vi "Top Level FPGA_LEDdebug.vi"() -> ()   [LabVIEW 2012]
uses:
  <vilib>/Platform/TimedLoop/XDataNode/timing_clust.ctl
  <vilib>/Platform/TimedLoop/XDataNode/nitl_modes.ctl
  <vilib>/Platform/TimedLoop/XDataNode/wakeup.ctl
  <vilib>/rvi/DataTransferAndStorage/Container/Common/niFpgaContainerMetaDataKey.ctl
  <vilib>/rvi/DataTransferAndStorage/Container/Common/niFpgaContainerState.ctl
  <vilib>/rvi/DataTransferAndStorage/Container/Common/niFpgaDataTypeControl.ctl
  <vilib>/rvi/DataTransferAndStorage/Container/Common/niFpgaContainerImplementationControl.ctl
  <vilib>/rvi/DataTransferAndStorage/Container/Common/niFpgaContainerArbitrationOptionsControl.ctl
  <vilib>/rvi/DataTransferAndStorage/Container/Common/niFpgaTransferTypeControl.ctl
  <vilib>/rvi/DataTransferAndStorage/Container/Common/niFpgaContainerInitializationParameters.ctl
  <vilib>/rvi/Memory/Memory_Types/niFpgaMemoryInterfaceConfiguration.ctl
  <vilib>/rvi/FIFO/Fifo_Types/niFpgaFifoControlLogicControl.ctl
  <vilib>/rvi/eio/common/nirviEmuTemplateMethod_errors.vi
  <vilib>/rvi/FIFO/Fifo_Resource/nirvififoEmulationSetSize.vi
  <vilib>/rvi/DataTransferAndStorage/Container/Common/niFpgaContainerGetUniqueNameForEmu.vi
  <vilib>/rvi/Emulation/niFpgaSctlEmulationRegisterWithScheduler.vi
  <vilib>/rvi/Emulation/niFpgaSctlEmulationScheduler.vi
  <vilib>/rvi/Emulation/niFpgaSctlEmulationFifoFullMgr.vi
  <vilib>/rvi/errors/niFpgaSetErrorForExecOnDevCompSimple.vi
  <vilib>/rvi/eio/common/nirviEmuReportErrorAndStop.vi
  <vilib>/rvi/Memory/Memory_Emulation/nirvimemoryEmulationManagerCache_GetValue.vi
  <vilib>/rvi/Memory/Memory_Emulation/niFpgaMemoryEmulationValidateCache.vi
  <vilib>/rvi/Memory/Memory_Emulation/nirvimemoryEmulationManagerCache_InsertValue.vi
  <vilib>/rvi/Memory/Memory_Emulation/nirvimemoryEmulationManagerCache_SetValue.vi
  <vilib>/rvi/Emulation/niFpgaSctlEmulationResourceMgr.vi
  <vilib>/rvi/Memory/Memory_Emulation/niFpgaMemoryEmulationCacheClearOnFirstRun.vi
  <vilib>/rvi/Memory/Memory_Emulation/nirvimemoryEmulationManagerCache_MakeExclusive.vi
  <vilib>/rvi/Memory/Memory_Emulation/nirvimemoryEmulationManagerCache_ReleaseExclusive.vi
  <vilib>/Utility/error.llb/Clear Errors.vi
  <vilib>/rvi/DataTransferAndStorage/Container/Common/niFpgaContainerSetEmuInfo.vi
  <vilib>/eio/EIONode/EIONode.xnode
  <vilib>/Platform/TimedLoop/XDataNode/XDataNode.xnode
  <vilib>/rvi/DataTransferAndStorage/Container/XNode/niFpgaContainer.xnode
  <vilib>/rvi/FIFO/Fifo_Resource/nirvififoEmulationClear.vi
  <vilib>/rvi/FIFO/Fifo_Resource/nirvififoEmulationRead.vi
  <vilib>/rvi/DataTransferAndStorage/Register/Emulation/niFpgaRegisterEmulation.vi
  <vilib>/rvi/Memory/Memory_Emulation/nirvimemoryEmulation.vi
  <vilib>/rvi/FIFO/Fifo_Resource/nirvififoEmulationWrite.vi
  <vilib>/rvi/LocalResourceManager/LocalResourceManager.xnode
  <vilib>/Platform/TimedLoop/XDataNode/XDNodeRunTimeDep.lvlib
panel:
  out "Total number of pulses sent":u64
  out "IO Module\\ADC Error A":bool
  out "IO Module\\ADC Error B":bool
  out "IO Module\\Pll Unlocked":bool
  out "Exited cleanly?":bool
  in  "Stop FPGA and exit":bool
  in  "Record Size only data":u32=95
  in  "show_trigger_position_for_debugging":bool
  out "DMA FIFO Timed Out?":bool
  in  "circular buffer length":u32=1000
  in  "location":i16(ring) items=["Purdue", "NIKHEF", "Zurich", "???"]
  in  "Trigger 0":i16=4000
  in  "Trigger 1":i16=4000
  in  "Trigger 2":i16=4000
  in  "Trigger 3":i16=4000
  in  "Trigger 4":i16=4000
  in  "Trigger 5":i16=4000
  in  "Trigger 6":i16=4000
  in  "Trigger 7":i16=4000
  in  "# of pretrigger":u32=20
  in  "initial value":u64
  in  "channel 0 on/off":bool
  in  "channel 2 on/off":bool
  in  "channel 1 on/off":bool
  in  "channel 3 on/off":bool
  in  "channel 4 on/off":bool
  in  "channel 5 on/off":bool
  in  "channel 6 on/off":bool
  in  "channel 7 on/off":bool
  in  "Testpulse duration (20 ns ticks)":u32=1
  in  "Testpulse Separation (20 ns ticks)":u32=50000
  in  "Testpulse Time Delay (20 ns ticks)":u32=15
  out "Timestamp":u64
  in  "Testpulser On/Off":bool
  out "Init Done":bool
  out "Initialize Flush DMA FIFO":bool
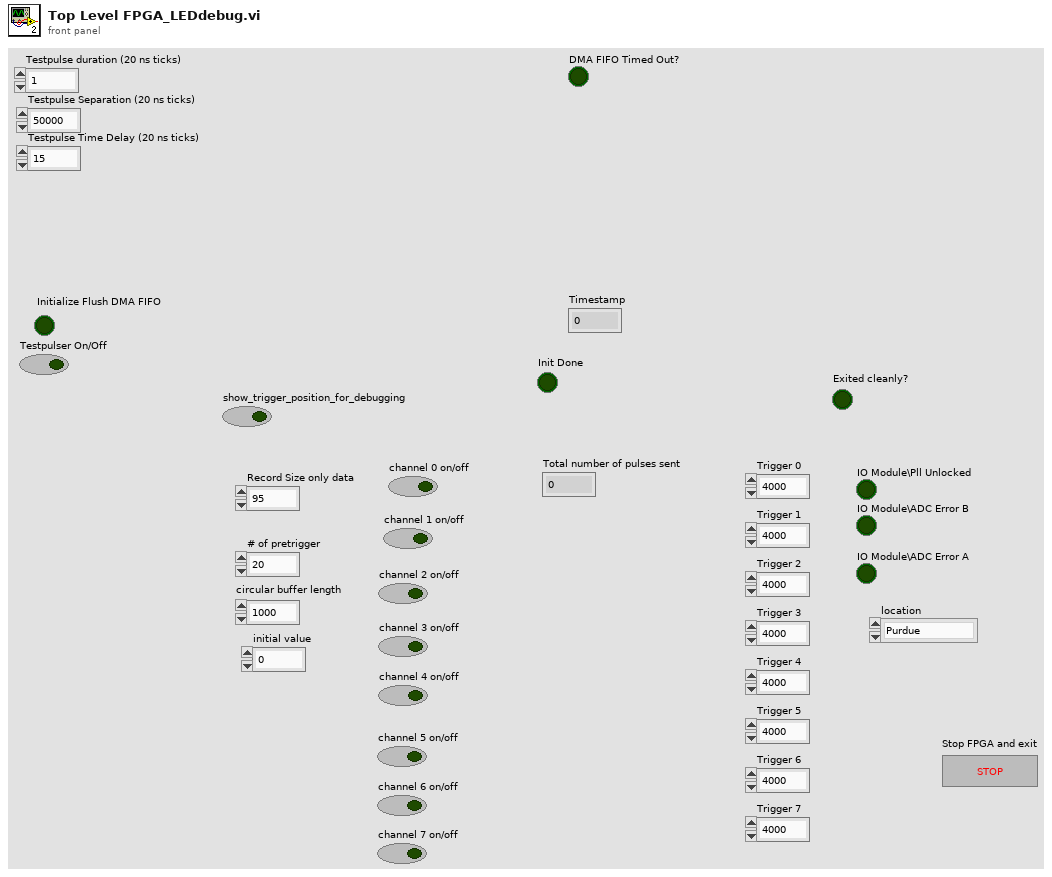
[diagram p1: front panel]
types:
  T1 = typedef "XDNodeRunTimeDep.lvlib/timing_clust.ctl" = cluster{"Expected End [f-1]":u64, "Actual End [f-1]":u64, "Finished Late? [f-1]":bool, "Expected End [i-1]":u64, "Actual End [i-1]":u64, "Finished Late? [i-1]":bool, "Expected Start [i]":u64, "Actual Start [i]":u64, "Expected Start [f]":u64, "Actual Start [f]":u64, "Source Name":string, "Structure Name":string, "Period":i64, "Deadline":i64, "Offset":i64, "Start":i64, "Priority":i32, "Timeout":i32, "Mode":T2, "Wakeup Reason":T3, "Error":errorcluster, "Source Type":string, "Secondary Source Type":string, "Global End Time":u64, "Global Start Time":u64, "Frame Duration":u64, "Iteration Duration":u64, "Assigned CPU":i32, "I/O Scan Engine Mode":u32}
  T2 = typedef "XDNodeRunTimeDep.lvlib/nitl_modes.ctl" = enum32{"No Change", "Process missed periods, maintain original phase", "Discard missed periods, maintain original phase", "Process missed periods, ignore original phase", "Discard missed periods, ignore original phase"}
  T3 = typedef "XDNodeRunTimeDep.lvlib/wakeup.ctl" = enum32{"Normal", "Aborted", "Asynchronous wakeup", "Timing source error", "Timed loop error", "Timeout"}
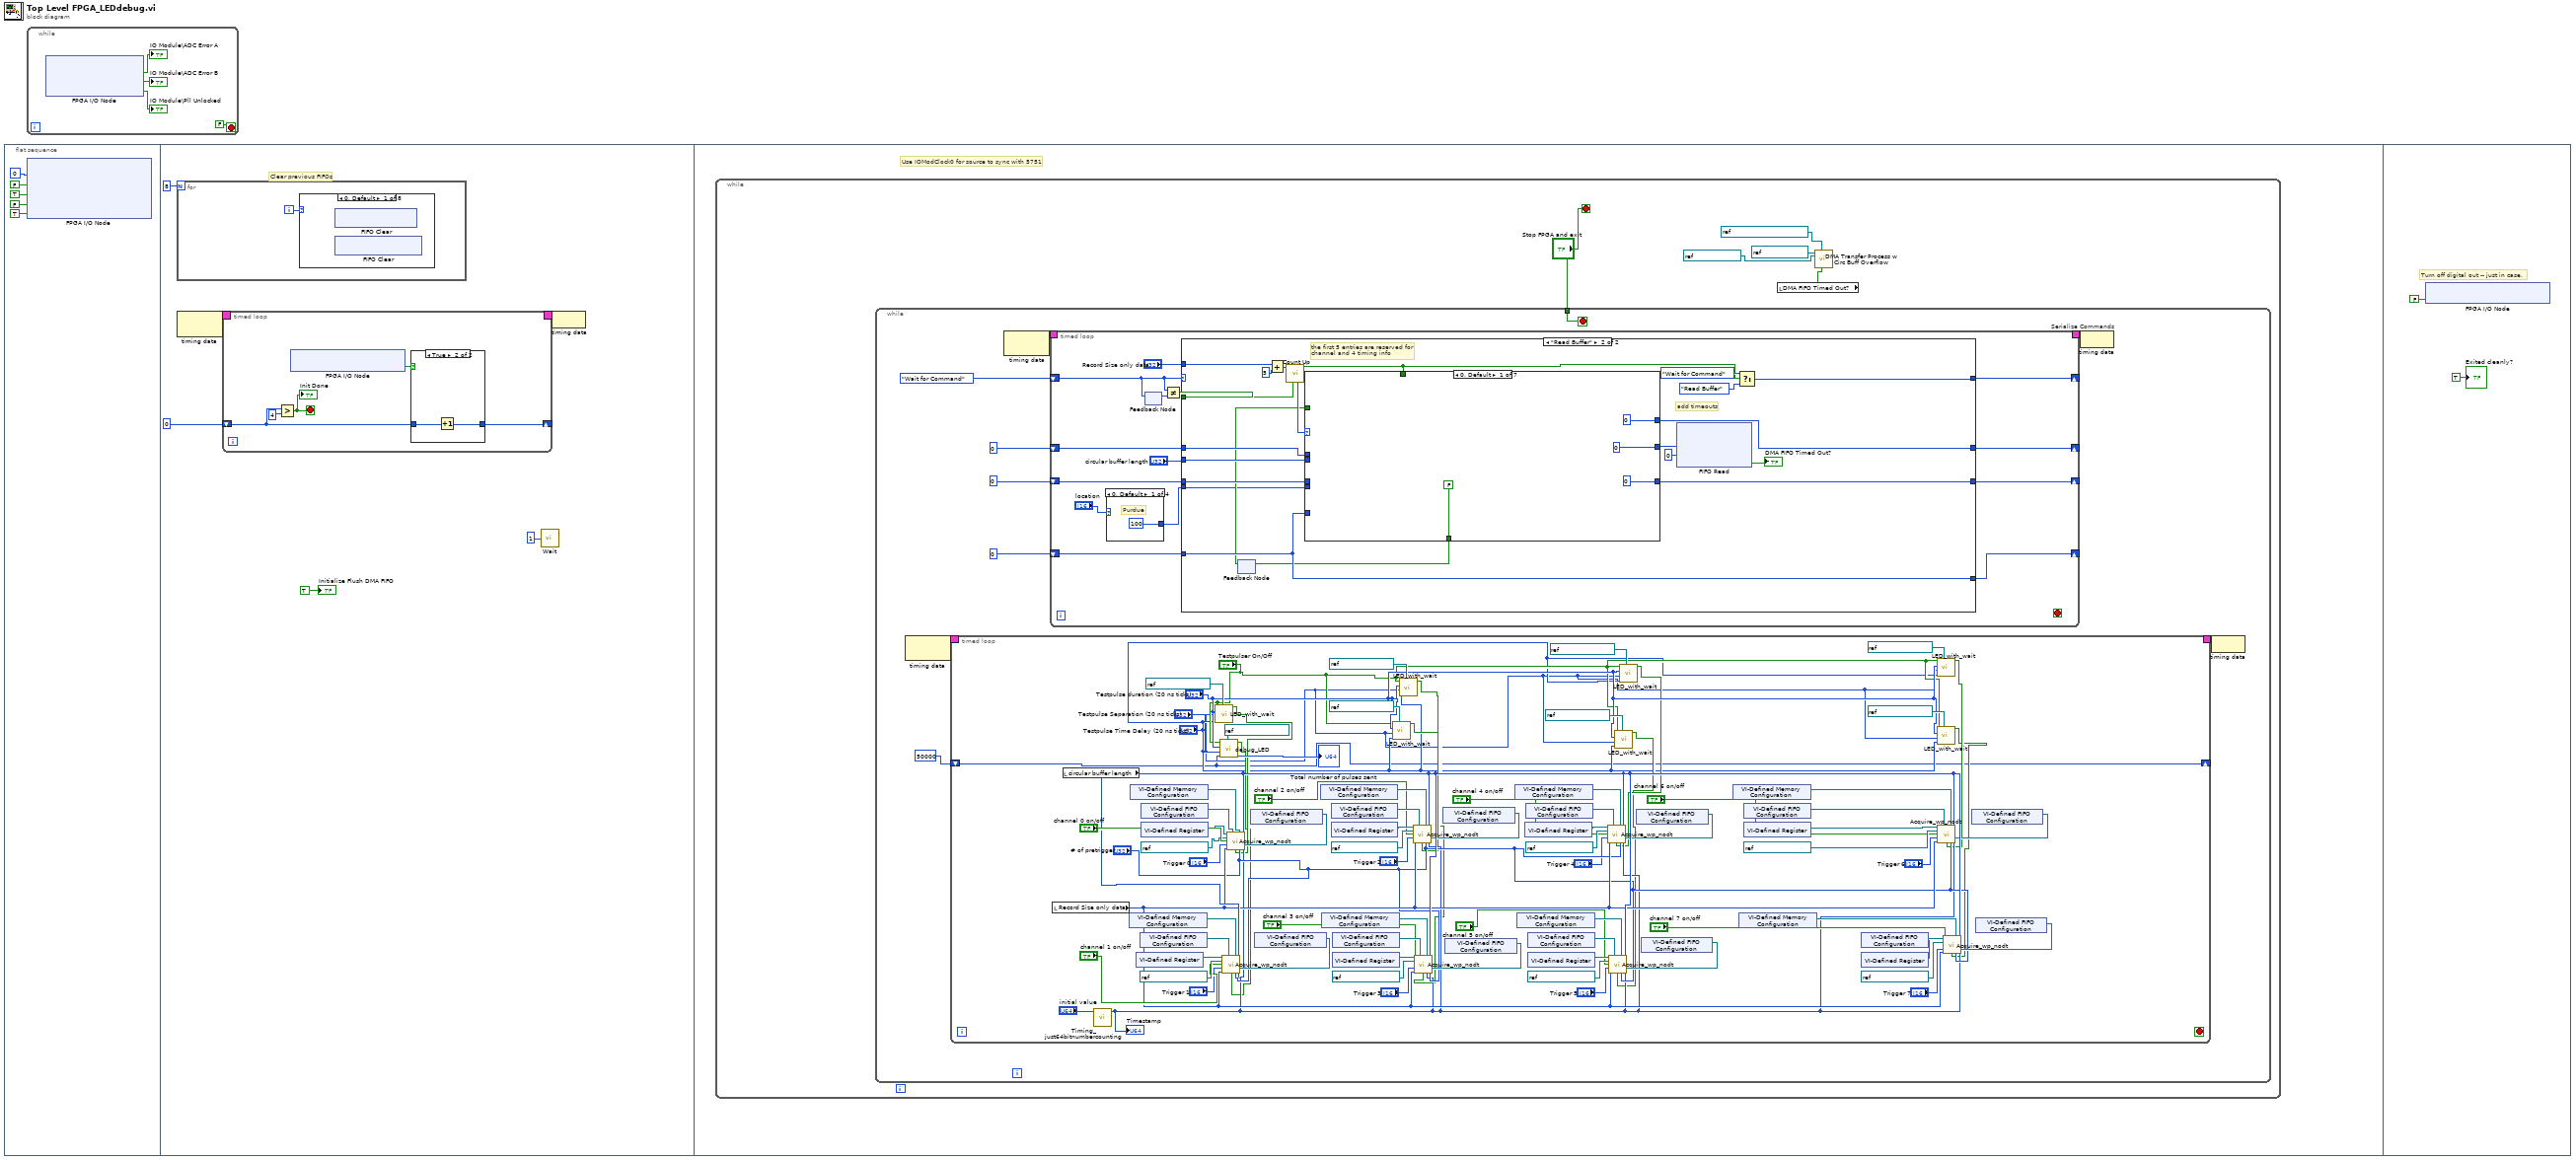
[diagram p0: block diagram]
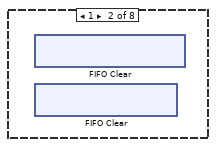
[diagram p2: hidden frame]
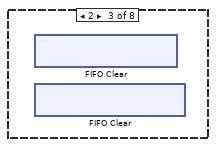
[diagram p3: hidden frame]
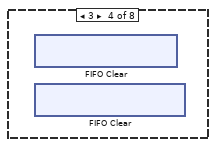
[diagram p4: hidden frame]
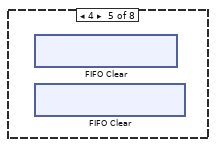
[diagram p5: hidden frame]
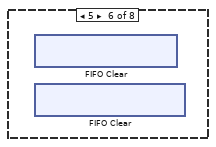
[diagram p6: hidden frame]
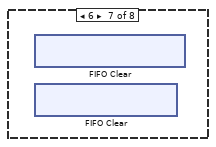
[diagram p7: hidden frame]
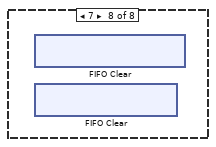
[diagram p8: hidden frame]
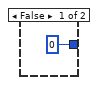
[diagram p9: hidden frame]
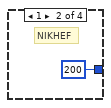
[diagram p10: hidden frame]
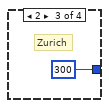
[diagram p11: hidden frame]
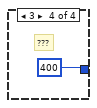
[diagram p12: hidden frame]
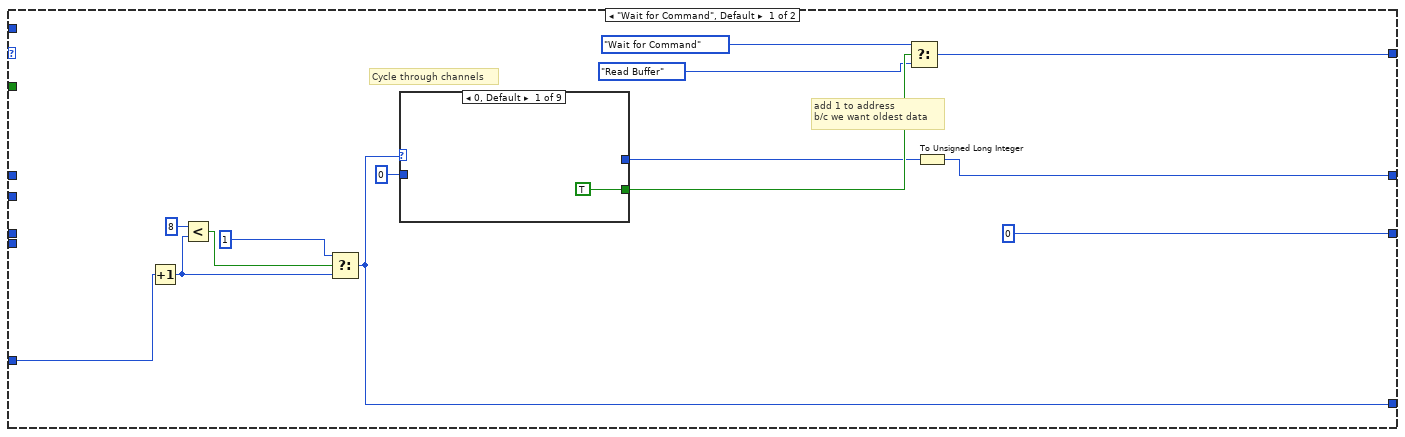
[diagram p13: hidden frame]
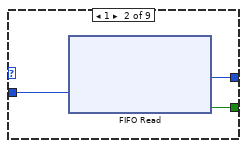
[diagram p14: hidden frame]
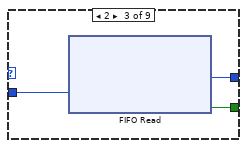
[diagram p15: hidden frame]
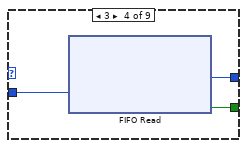
[diagram p16: hidden frame]
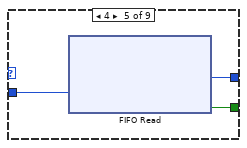
[diagram p17: hidden frame]
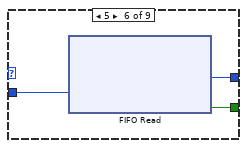
[diagram p18: hidden frame]
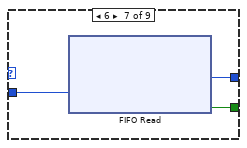
[diagram p19: hidden frame]
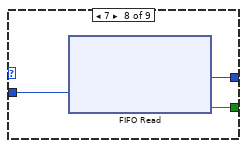
[diagram p20: hidden frame]
diagram:
  n1 = flat-sequence {
    frame #0 {
      n2 = xnode "FPGA I/O Node"("IO Module\\Sample Clock Select"=u8 0 ("IO Module\\Sample Clock Select"), "IO Module\\Force Initialization"=FALSE ("IO Module\\Force Initialization"), "IO Module\\Force Initialization"=TRUE ("IO Module\\Force Initialization"), "IO Module\\Force Initialization"=FALSE ("IO Module\\Force Initialization"), "IO Module\\Digital Output Enable"=TRUE ("IO Module\\Digital Output Enable")) -> ()  [unwired: 5 in, 5 out]
    }
    frame #1 {
      # "Clear previous FIFOs"
      n3 = for {
        N: 8 -> [_]
        i -> [w12]
        n4 = case shown="0, Default" w12 {
          frame 0, Default {
            n5 = xnode ("FIFO Clear")() -> ()  [unwired: 1 in, 1 out]
            n6 = xnode ("FIFO Clear")() -> ()  [unwired: 1 in, 1 out]
          }
          frame 1 {
            n7 = xnode ("FIFO Clear")() -> ()  [unwired: 1 in, 1 out]
            n8 = xnode ("FIFO Clear")() -> ()  [unwired: 1 in, 1 out]
          }
          frame 2 {
            n9 = xnode ("FIFO Clear")() -> ()  [unwired: 1 in, 1 out]
            n10 = xnode ("FIFO Clear")() -> ()  [unwired: 1 in, 1 out]
          }
          frame 3 {
            n11 = xnode ("FIFO Clear")() -> ()  [unwired: 1 in, 1 out]
            n12 = xnode ("FIFO Clear")() -> ()  [unwired: 1 in, 1 out]
          }
          frame 4 {
            n13 = xnode ("FIFO Clear")() -> ()  [unwired: 1 in, 1 out]
            n14 = xnode ("FIFO Clear")() -> ()  [unwired: 1 in, 1 out]
          }
          frame 5 {
            n15 = xnode ("FIFO Clear")() -> ()  [unwired: 1 in, 1 out]
            n16 = xnode ("FIFO Clear")() -> ()  [unwired: 1 in, 1 out]
          }
          frame 6 {
            n17 = xnode ("FIFO Clear")() -> ()  [unwired: 1 in, 1 out]
            n18 = xnode ("FIFO Clear")() -> ()  [unwired: 1 in, 1 out]
          }
          frame 7 {
            n19 = xnode ("FIFO Clear")() -> ()  [unwired: 1 in, 1 out]
            n20 = xnode ("FIFO Clear")() -> ()  [unwired: 1 in, 1 out]
          }
        }
      }
      n21 = node-c288() -> (w11:T1)  [unwired: 1 in]
      n22 = timed-loop {
        shift-right: [w16] -> _
        shift-left: u16 0 -> [w15]
        timing: w11 -> [_]
        timing-out: [_] -> w10
        stop <- w13 stop-if-true
        n23 = Greater?(x=w15, y=u16 4) -> (0:w13:bool)
        "Init Done" <- w13
        n24 = xnode "FPGA I/O Node"() -> ("IO Module\\Initialization Done"=w17:bool)  [unwired: 1 in, 1 out]
        n25 = case shown="True" w17 {
          tunnel: [u16 0 w20] -> w16
          tunnel: w15 -> [_ w19]
          frame False {
          }
          frame True {
            n26 = Increment(x=w19) -> (x+1=w20:u16)
          }
        }
      }
      n27 = call "Wait"("Count(mSec)"=u32 1) -> ()  [unwired: 1 out]
      n28 = node-c288(w10) -> ()
      "Initialize Flush DMA FIFO" <- TRUE ("Initialize Flush DMA FIFO")
    }
    frame #2 {
      # "Use IOModClock0 for source to sync with 5751"
      n29 = while {
        stop <- "Stop FPGA and exit" stop-if-true
        n30 = while {
          tunnel: "Stop FPGA and exit" -> [w31]
          stop <- w31 stop-if-true
          n31 = node-c288() -> (w37:T1)  [unwired: 1 in]
          n32 = timed-loop {
            timing: w37 -> [_]
            timing-out: [_] -> w36
            shift-right: [w40] -> _
            shift-left: u32 50000 ("Testpulse Separation (20 ns ticks) 3") -> [w40]
            stop <- _ stop-if-true
            n33 = local read "Record Size only data"() -> (w82:u32)
            n34 = local read "circular buffer length"() -> (w83:u32)
            n35 = call "Timing_just64bitnumbercounting.vi"("initial value"="initial value") -> ("x+1"=w54:u64)  [unwired: 10 in]
            "Timestamp" <- w54
            n36 = xnode "VI-Defined Memory Configuration"() -> ("Memory Out"=w122:refnum<k21>)
            n37 = xnode "VI-Defined Memory Configuration"() -> ("Memory Out"=w84:refnum<k21>)
            n38 = xnode "VI-Defined Register"() -> ("Register Out"=w78:refnum<k21>)
            n39 = xnode "VI-Defined FIFO Configuration"() -> ("FIFO Out"=w121:refnum<k21>)
            n40 = xnode "VI-Defined FIFO Configuration"() -> ("FIFO Out"=w85:refnum<k21>)
            n41 = xnode "VI-Defined Register"() -> ("Register Out"=w79:refnum<k21>)
            n42 = call "LED_with_wait.vi"("FPGA I/O In"=refnum<k21> "IO Module\\D0 0", "Testpulse Time Delay (20 ns ticks)"="Testpulse Time Delay (20 ns ticks)", "Testpulse Separation (20 ns ticks)"="Testpulse Separation (20 ns ticks)", "Testpulse duration (20 ns ticks)"="Testpulse duration (20 ns ticks)", "Testpulser On/Off"="Testpulser On/Off") -> ("Is Test Pulse?"=w50:bool)  [unwired: 4 in, 2 out]
            n43 = call "debug_LED.vi"("FPGA I/O In"=refnum<k21> "IO Module\\D0 1", "Test pulse separation (20 ns ticks)"=w40, "Testpulse Time Delay (20 ns ticks)"="Testpulse Time Delay (20 ns ticks)", "Testpulse duration (20 ns ticks)"="Testpulse duration (20 ns ticks)", "Testpulser On/Off"="Testpulser On/Off") -> ("Total number of pulses sent"=→"Total number of pulses sent":u64, "Is Test Pulse?"=w49:bool)  [unwired: 5 in]
            n44 = xnode "VI-Defined FIFO Configuration"() -> ("FIFO Out"=w71:refnum<k21>)
            n45 = call "Acquire_wp_nodt.vi"("Ch Armed Reg"=w79, "Command FIFO"=w85, "Circular Buffer Mem"=w84, "circular buffer length"=w83, "FPGA I/O In"=refnum<k21> "IO Module\\AI A0", "channel on/off"="channel 0 on/off", "Trigger"="Trigger 0", "Timing FIFO"=w71, "Samples to Acquire"=w82, "Is Test Pulse?"=w50, "# of pretrigger"="# of pretrigger", "timing"=w54) -> ()  [unwired: 4 in]
            n46 = xnode "VI-Defined FIFO Configuration"() -> ("FIFO Out"=w64:refnum<k21>)
            n47 = call "Acquire_wp_nodt.vi"("Ch Armed Reg"=w78, "Command FIFO"=w121, "Circular Buffer Mem"=w122, "circular buffer length"=w83, "FPGA I/O In"=refnum<k21> "IO Module\\AI A1", "channel on/off"="channel 1 on/off", "Trigger"="Trigger 1", "Timing FIFO"=w64, "Samples to Acquire"=w82, "Is Test Pulse?"=w49, "# of pretrigger"="# of pretrigger", "timing"=w54) -> ()  [unwired: 4 in]
            n48 = xnode "VI-Defined Memory Configuration"() -> ("Memory Out"=w118:refnum<k21>)
            n49 = xnode "VI-Defined Memory Configuration"() -> ("Memory Out"=w119:refnum<k21>)
            n50 = xnode "VI-Defined FIFO Configuration"() -> ("FIFO Out"=w117:refnum<k21>)
            n51 = xnode "VI-Defined Register"() -> ("Register Out"=w105:refnum<k21>)
            n52 = xnode "VI-Defined FIFO Configuration"() -> ("FIFO Out"=w120:refnum<k21>)
            n53 = xnode "VI-Defined Register"() -> ("Register Out"=w107:refnum<k21>)
            n54 = call "LED_with_wait.vi"("FPGA I/O In"=refnum<k21> "IO Module\\D0 3", "Testpulse Time Delay (20 ns ticks)"="Testpulse Time Delay (20 ns ticks)", "Testpulse Separation (20 ns ticks)"="Testpulse Separation (20 ns ticks)", "Testpulse duration (20 ns ticks)"="Testpulse duration (20 ns ticks)", "Testpulser On/Off"="Testpulser On/Off") -> ("Is Test Pulse?"=w47:bool)  [unwired: 4 in, 2 out]
            n55 = call "LED_with_wait.vi"("FPGA I/O In"=refnum<k21> "IO Module\\D0 2", "Testpulse Time Delay (20 ns ticks)"="Testpulse Time Delay (20 ns ticks)", "Testpulse Separation (20 ns ticks)"="Testpulse Separation (20 ns ticks)", "Testpulse duration (20 ns ticks)"="Testpulse duration (20 ns ticks)", "Testpulser On/Off"="Testpulser On/Off") -> ("Is Test Pulse?"=w48:bool)  [unwired: 4 in, 2 out]
            n56 = xnode "VI-Defined FIFO Configuration"() -> ("FIFO Out"=w70:refnum<k21>)
            n57 = call "Acquire_wp_nodt.vi"("Ch Armed Reg"=w105, "Command FIFO"=w117, "Circular Buffer Mem"=w118, "circular buffer length"=w83, "FPGA I/O In"=refnum<k21> "IO Module\\AI A2", "channel on/off"="channel 2 on/off", "Trigger"="Trigger 2", "Timing FIFO"=w70, "Samples to Acquire"=w82, "Is Test Pulse?"=w48, "# of pretrigger"="# of pretrigger", "timing"=w54) -> ()  [unwired: 4 in]
            n58 = xnode "VI-Defined FIFO Configuration"() -> ("FIFO Out"=w65:refnum<k21>)
            n59 = call "Acquire_wp_nodt.vi"("Ch Armed Reg"=w107, "Command FIFO"=w120, "Circular Buffer Mem"=w119, "circular buffer length"=w83, "FPGA I/O In"=refnum<k21> "IO Module\\AI A3", "channel on/off"="channel 3 on/off", "Trigger"="Trigger 3", "Timing FIFO"=w65, "Samples to Acquire"=w82, "Is Test Pulse?"=w47, "# of pretrigger"="# of pretrigger", "timing"=w54) -> ()  [unwired: 4 in]
            n60 = xnode "VI-Defined Memory Configuration"() -> ("Memory Out"=w110:refnum<k21>)
            n61 = xnode "VI-Defined Memory Configuration"() -> ("Memory Out"=w111:refnum<k21>)
            n62 = xnode "VI-Defined Register"() -> ("Register Out"=w99:refnum<k21>)
            n63 = xnode "VI-Defined FIFO Configuration"() -> ("FIFO Out"=w109:refnum<k21>)
            n64 = xnode "VI-Defined FIFO Configuration"() -> ("FIFO Out"=w112:refnum<k21>)
            n65 = xnode "VI-Defined Register"() -> ("Register Out"=w103:refnum<k21>)
            n66 = call "LED_with_wait.vi"("FPGA I/O In"=refnum<k21> "IO Module\\D0 5", "Testpulse Time Delay (20 ns ticks)"="Testpulse Time Delay (20 ns ticks)", "Testpulse Separation (20 ns ticks)"="Testpulse Separation (20 ns ticks)", "Testpulse duration (20 ns ticks)"="Testpulse duration (20 ns ticks)", "Testpulser On/Off"="Testpulser On/Off") -> ("Is Test Pulse?"=w45:bool)  [unwired: 4 in, 2 out]
            n67 = call "LED_with_wait.vi"("FPGA I/O In"=refnum<k21> "IO Module\\D0 4", "Testpulse Time Delay (20 ns ticks)"="Testpulse Time Delay (20 ns ticks)", "Testpulse Separation (20 ns ticks)"="Testpulse Separation (20 ns ticks)", "Testpulse duration (20 ns ticks)"="Testpulse duration (20 ns ticks)", "Testpulser On/Off"="Testpulser On/Off") -> ("Is Test Pulse?"=w46:bool)  [unwired: 4 in, 2 out]
            n68 = xnode "VI-Defined FIFO Configuration"() -> ("FIFO Out"=w69:refnum<k21>)
            n69 = call "Acquire_wp_nodt.vi"("Ch Armed Reg"=w99, "Command FIFO"=w109, "Circular Buffer Mem"=w110, "circular buffer length"=w83, "FPGA I/O In"=refnum<k21> "IO Module\\AI A4", "channel on/off"="channel 4 on/off", "Trigger"="Trigger 4", "Timing FIFO"=w69, "Samples to Acquire"=w82, "Is Test Pulse?"=w46, "# of pretrigger"="# of pretrigger", "timing"=w54) -> ()  [unwired: 4 in]
            n70 = xnode "VI-Defined FIFO Configuration"() -> ("FIFO Out"=w66:refnum<k21>)
            n71 = call "Acquire_wp_nodt.vi"("Ch Armed Reg"=w103, "Command FIFO"=w112, "Circular Buffer Mem"=w111, "circular buffer length"=w83, "FPGA I/O In"=refnum<k21> "IO Module\\AI A5", "channel on/off"="channel 5 on/off", "Trigger"="Trigger 5", "Timing FIFO"=w66, "Samples to Acquire"=w82, "Is Test Pulse?"=w45, "# of pretrigger"="# of pretrigger", "timing"=w54) -> ()  [unwired: 4 in]
            n72 = xnode "VI-Defined Memory Configuration"() -> ("Memory Out"=w115:refnum<k21>)
            n73 = xnode "VI-Defined Memory Configuration"() -> ("Memory Out"=w114:refnum<k21>)
            n74 = xnode "VI-Defined FIFO Configuration"() -> ("FIFO Out"=w116:refnum<k21>)
            n75 = xnode "VI-Defined Register"() -> ("Register Out"=w101:refnum<k21>)
            n76 = xnode "VI-Defined FIFO Configuration"() -> ("FIFO Out"=w113:refnum<k21>)
            n77 = xnode "VI-Defined Register"() -> ("Register Out"=w97:refnum<k21>)
            n78 = call "LED_with_wait.vi"("FPGA I/O In"=refnum<k21> "IO Module\\D0 6", "Testpulse Time Delay (20 ns ticks)"="Testpulse Time Delay (20 ns ticks)", "Testpulse Separation (20 ns ticks)"="Testpulse Separation (20 ns ticks)", "Testpulse duration (20 ns ticks)"="Testpulse duration (20 ns ticks)", "Testpulser On/Off"="Testpulser On/Off") -> ("Is Test Pulse?"=w44:bool)  [unwired: 4 in, 2 out]
            n79 = call "LED_with_wait.vi"("FPGA I/O In"=refnum<k21> "IO Module\\D0 7", "Testpulse Time Delay (20 ns ticks)"="Testpulse Time Delay (20 ns ticks)", "Testpulse Separation (20 ns ticks)"="Testpulse Separation (20 ns ticks)", "Testpulse duration (20 ns ticks)"="Testpulse duration (20 ns ticks)", "Testpulser On/Off"="Testpulser On/Off") -> ("Is Test Pulse?"=w43:bool)  [unwired: 4 in, 2 out]
            n80 = xnode "VI-Defined FIFO Configuration"() -> ("FIFO Out"=w68:refnum<k21>)
            n81 = call "Acquire_wp_nodt.vi"("Ch Armed Reg"=w101, "Command FIFO"=w116, "Circular Buffer Mem"=w115, "circular buffer length"=w83, "FPGA I/O In"=refnum<k21> "IO Module\\AI A6", "channel on/off"="channel 6 on/off", "Trigger"="Trigger 6", "Timing FIFO"=w68, "Samples to Acquire"=w82, "Is Test Pulse?"=w44, "# of pretrigger"="# of pretrigger", "timing"=w54) -> ()  [unwired: 4 in]
            n82 = xnode "VI-Defined FIFO Configuration"() -> ("FIFO Out"=w67:refnum<k21>)
            n83 = call "Acquire_wp_nodt.vi"("Ch Armed Reg"=w97, "Command FIFO"=w113, "Circular Buffer Mem"=w114, "circular buffer length"=w83, "FPGA I/O In"=refnum<k21> "IO Module\\AI A7", "channel on/off"="channel 7 on/off", "Trigger"="Trigger 7", "Timing FIFO"=w67, "Samples to Acquire"=w82, "Is Test Pulse?"=w43, "# of pretrigger"="# of pretrigger", "timing"=w54) -> ()  [unwired: 4 in]
          }
          n84 = node-c288() -> (w39:T1)  [unwired: 1 in]
          n85 = timed-loop "Serialize Commands" {
            timing: w39 -> [_]
            timing-out: [_] -> w38
            shift-right: [w903] -> _
            shift-left: enum16{"Wait for Command", "Read Buffer"}."Wait for Command" -> [w901]
            shift-right: [w907] -> _
            shift-left: u32 0 ("Element") -> [w906]
            shift-right: [w905] -> _
            shift-left: u8 0 ("t") -> [w904]
            shift-right: [w898] -> _
            shift-left: u64 0 ("Element") -> [w897]
            stop <- _ stop-if-true
            n86 = case shown="0, Default" "location" {
              tunnel: [i16 100 i16 200 i16 300 i16 400] -> w895
              frame 0, Default {
                # "Purdue"
              }
              frame 1 {
                # "NIKHEF"
              }
              frame 2 {
                # "Zurich"
              }
              frame 3 {
                # "???"
              }
            }
            n87 = feedback-in #1(w901) -> ()
            n88 = feedback #1() -> (w902:enum16{"Wait for Command", "Read Buffer"})  [unwired: 1 in]
            n89 = Not Equal?(x=w901, y=w902) -> (x != y?=w899:bool)
            n90 = case shown="\"Read Buffer\"" w901 {
              tunnel: "Record Size only data" -> [_ w961]
              tunnel: [w915 w971] -> w905
              tunnel: w904 -> [w917 w971]
              tunnel: [w918 w956] -> w907
              tunnel: w906 -> [_ w970]
              tunnel: [w921 w972] -> w903
              tunnel: "circular buffer length" -> [_ w969]
              tunnel: w899 -> [_ w963]
              tunnel: [u64 0 ("Element") w958] -> w898
              tunnel: w897 -> [_ w957]
              tunnel: w895 -> [_ w952]
              frame "Wait for Command", Default {
                # "add 1 to address\nb/c we want oldest data"
                # "Cycle through channels"
                n91 = Increment(x=w917) -> (x+1=w916:u8)
                n92 = Less?(x=u8 8, y=w916) -> (x < y?=w925:bool)
                n93 = Select(t=u8 1, s=w925, f=w916) -> (s? t:f=w915:u8)
                n94 = case shown="0, Default" w915 {
                  tunnel: [TRUE ("Timed Out?") w930 w931 w934 w937 w940 w943 w946 w949] -> w922
                  tunnel: 0 ("Timeout") -> [_ w929 w933 w936 w939 w942 w945 w948 w951]
                  tunnel: [_ w928 w932 w935 w938 w941 w944 w947 w950] -> w914
                  frame 0, Default {
                  }
                  frame 1 {
                    n95 = xnode ("FIFO Read")("Timeout"=w929) -> ("Element"=w928:i16, "Timed Out?"=w930:bool)  [unwired: 1 in, 1 out]
                  }
                  frame 2 {
                    n96 = xnode ("FIFO Read")("Timeout"=w933) -> ("Element"=w932:i16, "Timed Out?"=w931:bool)  [unwired: 1 in, 1 out]
                  }
                  frame 3 {
                    n97 = xnode ("FIFO Read")("Timeout"=w936) -> ("Element"=w935:i16, "Timed Out?"=w934:bool)  [unwired: 1 in, 1 out]
                  }
                  frame 4 {
                    n98 = xnode ("FIFO Read")("Timeout"=w939) -> ("Element"=w938:i16, "Timed Out?"=w937:bool)  [unwired: 1 in, 1 out]
                  }
                  frame 5 {
                    n99 = xnode ("FIFO Read")("Timeout"=w942) -> ("Element"=w941:i16, "Timed Out?"=w940:bool)  [unwired: 1 in, 1 out]
                  }
                  frame 6 {
                    n100 = xnode ("FIFO Read")("Timeout"=w945) -> ("Element"=w944:i16, "Timed Out?"=w943:bool)  [unwired: 1 in, 1 out]
                  }
                  frame 7 {
                    n101 = xnode ("FIFO Read")("Timeout"=w948) -> ("Element"=w947:i16, "Timed Out?"=w946:bool)  [unwired: 1 in, 1 out]
                  }
                  frame 8 {
                    n102 = xnode ("FIFO Read")("Timeout"=w951) -> ("Element"=w950:i16, "Timed Out?"=w949:bool)  [unwired: 1 in, 1 out]
                  }
                }
                n103 = Select(t=enum16{"Wait for Command", "Read Buffer"}."Wait for Command", s=w922, f=enum16{"Wait for Command", "Read Buffer"}."Read Buffer") -> (s? t:f=w921:enum16{"Wait for Command", "Read Buffer"})
                n104 = To Unsigned Long Integer(number=w914) -> (unsigned 32bit integer=w918:u32)
              }
              frame "Read Buffer" {
                # "the first 5 entries are reserved for channel and 4 timing info"
                # "add timeouts"
                n105 = feedback #2() -> (w955:bool)  [unwired: 1 in]
                n106 = Add(x=w961, y=u32 5) -> (x+y=w959:u32)
                n107 = call "Count Up.vi"("Reset?"=w963, "goal"=w959) -> ("Count Met"=w965:bool, "count"=w962:u32)  [unwired: 8 in]
                n108 = case shown="0, Default" w962 {
                  tunnel: w971 -> [_ w981 w986 _ _ _ w1034]
                  tunnel: w970 -> [_ w985 w988 w1018 w1024 w1030 w1041]
                  tunnel: w969 -> [_ _ _ _ _ _ w1040]
                  tunnel: w965 -> [_ _ _ _ _ _ w1039]
                  tunnel: [i16 0 ("Data") w982 w992 w1016 w1022 w1028 w1035] -> w964
                  tunnel: w955 -> [_ _ _ _ _ _ w1037]
                  tunnel: [u64 0 ("Element") _ w991 w1019 w1025 w1031 _] -> w958
                  tunnel: w957 -> [_ _ _ w1019 w1025 w1031 _]
                  tunnel: [u32 0 ("Element") w985 w988 w1018 w1024 w1030 _] -> w956
                  tunnel: [FALSE FALSE FALSE FALSE FALSE TRUE FALSE] -> w954
                  tunnel: w952 -> [_ w977 _ _ _ _ _]
                  frame 0, Default {
                  }
                  frame 1 {
                    w983 = u16 0 items=["Header Information", "Particle Pulse", "Test Pulse"] ("Pulse Type")
                    n109 = Decrement(x=w981) -> (x-1=w980:u8)
                    n110 = To Word Integer(number=w980) -> (16bit integer=w979:i16)
                    n111 = Add(x=w977, y=w979) -> (x+y=w978:i16)
                    n112 = call "bitmanip.vi"("Pulse Type"=w983, "Integer to be written"=w978) -> ("Integer Written"=w982:i16)  [unwired: 2 in]
                  }
                  frame 2 {
                    n113 = case shown="1" w986 {
                      tunnel: [_ w993 w995 w997 w999 w1001 w1003 w1005 w1007] -> w987
                      frame Default {
                      }
                      frame 1 {
                        n114 = xnode ("FIFO Read")("Timeout"=0) -> ("Element"=w993:u64)  [unwired: 1 in, 2 out]
                      }
                      frame 2 {
                        n115 = xnode ("FIFO Read")("Timeout"=0) -> ("Element"=w995:u64)  [unwired: 1 in, 2 out]
                      }
                      frame 3 {
                        n116 = xnode ("FIFO Read")("Timeout"=0) -> ("Element"=w997:u64)  [unwired: 1 in, 2 out]
                      }
                      frame 4 {
                        n117 = xnode ("FIFO Read")("Timeout"=0) -> ("Element"=w999:u64)  [unwired: 1 in, 2 out]
                      }
                      frame 5 {
                        n118 = xnode ("FIFO Read")("Timeout"=0) -> ("Element"=w1001:u64)  [unwired: 1 in, 2 out]
                      }
                      frame 6 {
                        n119 = xnode ("FIFO Read")("Timeout"=0) -> ("Element"=w1003:u64)  [unwired: 1 in, 2 out]
                      }
                      frame 7 {
                        n120 = xnode ("FIFO Read")("Timeout"=0) -> ("Element"=w1005:u64)  [unwired: 1 in, 2 out]
                      }
                      frame 8 {
                        n121 = xnode ("FIFO Read")("Timeout"=0) -> ("Element"=w1007:u64)  [unwired: 1 in, 2 out]
                      }
                    }
                    n122 = case shown="True" "show_trigger_position_for_debugging" {
                      tunnel: [w1009 w1013] -> w992
                      tunnel: [w1011 w1014] -> w991
                      tunnel: w988 -> [_ w1015]
                      tunnel: w987 -> [w1011 w1014]
                      frame False {
                        # "reads out the lsb of the timing information"
                        n123 = Split Number(x=w1011) -> (hi(x)=w1012:u32)  [unwired: 1 out]
                        n124 = Split Number(x=w1012) -> (hi(x)=w1010:u16)  [unwired: 1 out]
                        n125 = To Word Integer(number=w1010) -> (16bit integer=w1009:i16)
                      }
                      frame True {
                        # "plot trigger position instead of the first timing bin"
                        n126 = To Word Integer(number=w1015) -> (16bit integer=w1013:i16)
                      }
                    }
                  }
                  frame 3 {
                    n127 = Split Number(x=w1019) -> (hi(x)=w1021:u32)  [unwired: 1 out]
                    n128 = Split Number(x=w1021) -> (lo(x)=w1020:u16)  [unwired: 1 out]
                    n129 = To Word Integer(number=w1020) -> (16bit integer=w1016:i16)
                  }
                  frame 4 {
                    n130 = Split Number(x=w1025) -> (lo(x)=w1027:u32)  [unwired: 1 out]
                    n131 = Split Number(x=w1027) -> (hi(x)=w1026:u16)  [unwired: 1 out]
                    n132 = To Word Integer(number=w1026) -> (16bit integer=w1022:i16)
                  }
                  frame 5 {
                    n133 = Split Number(x=w1031) -> (lo(x)=w1033:u32)  [unwired: 1 out]
                    n134 = Split Number(x=w1033) -> (lo(x)=w1032:u16)  [unwired: 1 out]
                    n135 = To Word Integer(number=w1032) -> (16bit integer=w1028:i16)
                  }
                  frame 6.. {
                    n136 = call "Circular Buffer Address_try_without_deadtime.vi"("Reset?"=w1037, "Starting Address"=w1041, "circular buffer length"=w1040) -> ("Address"=w1038:u32)  [unwired: 8 in]
                    n137 = case shown="Default" w1034 {
                      tunnel: w1038 -> [_ w1045 w1048 w1051 w1054 w1057 w1060 w1063 w1066]
                      tunnel: w1039 -> [_ w1044 w1047 w1050 w1053 w1056 w1059 w1062 w1065]
                      tunnel: [i16 0 w1043 w1046 w1049 w1052 w1055 w1058 w1061 w1064] -> w1035
                      frame Default {
                        # "Error"
                      }
                      frame 1 {
                        n138 = xnode ("Memory Read")("Address"=w1045) -> ("Data"=w1043:i16)  [unwired: 1 in, 1 out]
                        n139 = xnode ("Register Write")("Data"=w1044) -> ()  [unwired: 1 in, 1 out]
                      }
                      frame 2 {
                        n140 = xnode ("Memory Read")("Address"=w1048) -> ("Data"=w1046:i16)  [unwired: 1 in, 1 out]
                        n141 = xnode ("Register Write")("Data"=w1047) -> ()  [unwired: 1 in, 1 out]
                      }
                      frame 3 {
                        n142 = xnode ("Memory Read")("Address"=w1051) -> ("Data"=w1049:i16)  [unwired: 1 in, 1 out]
                        n143 = xnode ("Register Write")("Data"=w1050) -> ()  [unwired: 1 in, 1 out]
                      }
                      frame 4 {
                        n144 = xnode ("Memory Read")("Address"=w1054) -> ("Data"=w1052:i16)  [unwired: 1 in, 1 out]
                        n145 = xnode ("Register Write")("Data"=w1053) -> ()  [unwired: 1 in, 1 out]
                      }
                      frame 5 {
                        n146 = xnode ("Memory Read")("Address"=w1057) -> ("Data"=w1055:i16)  [unwired: 1 in, 1 out]
                        n147 = xnode ("Register Write")("Data"=w1056) -> ()  [unwired: 1 in, 1 out]
                      }
                      frame 6 {
                        n148 = xnode ("Memory Read")("Address"=w1060) -> ("Data"=w1058:i16)  [unwired: 1 in, 1 out]
                        n149 = xnode ("Register Write")("Data"=w1059) -> ()  [unwired: 1 in, 1 out]
                      }
                      frame 7 {
                        n150 = xnode ("Memory Read")("Address"=w1063) -> ("Data"=w1061:i16)  [unwired: 1 in, 1 out]
                        n151 = xnode ("Register Write")("Data"=w1062) -> ()  [unwired: 1 in, 1 out]
                      }
                      frame 8 {
                        n152 = xnode ("Memory Read")("Address"=w1066) -> ("Data"=w1064:i16)  [unwired: 1 in, 1 out]
                        n153 = xnode ("Register Write")("Data"=w1065) -> ()  [unwired: 1 in, 1 out]
                      }
                    }
                  }
                }
                n154 = feedback-in #2(w954) -> ()
                n155 = xnode ("FIFO Read")("Element"=w964, "Timeout"=0) -> ("Timed Out?"=→"DMA FIFO Timed Out?":bool)  [unwired: 1 in, 1 out]
                n156 = Select(t=enum16{"Wait for Command", "Read Buffer"}."Wait for Command", s=w965, f=enum16{"Wait for Command", "Read Buffer"}."Read Buffer") -> (s? t:f=w972:enum16{"Wait for Command", "Read Buffer"})
              }
            }
          }
          n157 = node-c288(w38) -> ()
          n158 = node-c288(w36) -> ()
        }
        n159 = local read "DMA FIFO Timed Out?"() -> (w26:bool)
        n160 = call "DMA Transfer Process w Circ Buff Overflow.vi"("DMA Write Timed Out?"=w26, "Clock Domain"=refnum<k21> "40 MHz Onboard Clock", "Local"=refnum<k21> "To DMA FIFO", "DMA"=refnum<k21> "To Host FIFO") -> ()  [unwired: 8 in]
      }
    }
    frame #3 {
      # "Turn off digital out -- just in case."
      n161 = xnode "FPGA I/O Node"("IO Module\\Digital Output Enable"=FALSE ("IO Module\\Digital Output Enable")) -> ()  [unwired: 1 in, 1 out]
      "Exited cleanly?" <- TRUE ("Exited cleanly?")
    }
  }
  n162 = while {
    stop <- FALSE stop-if-true
    n163 = xnode "FPGA I/O Node"() -> ("IO Module\\ADC Error A"=→"IO Module\\ADC Error A":bool, "IO Module\\ADC Error B"=→"IO Module\\ADC Error B":bool, "IO Module\\Pll Unlocked"=→"IO Module\\Pll Unlocked":bool)  [unwired: 3 in, 3 out]
  }
